vi "PWM Input Post Step.vi"(8 "error in (no error)":errorcluster, 9 "PWM Input In":T1, 10 "Socket No":u16=1, 11 "NI PWM Input in":refnum<class "NI PWM Input.lvclass">) -> (0 "error out":errorcluster, 1 "Frequency":dbl[](array[numeric]), 2 "Report Text":string, 3 "NI PWM Input out":refnum<class "NI PWM Input.lvclass">, 4 "Duty Cycle":dbl[](array[numeric]), 5 "Physical Channel":string[](array[string]))   [LabVIEW 2023, in "HardwareAbstractionLayer_LVOOP.lvlib" / "NI PWM Input.lvclass"]
uses:
  NI PWM Input.lvclass
  Control/PWMInputEdit.ctl
  NI PWM Input.lvclass/NI PWM Input.ctl
  Database/Database.lvclass
  <resource>/objmgr/daqmx.rc
panel:
  out "PhysicalChans":tag[](array[tag])
  out "CounterName":tag[](array[tag])
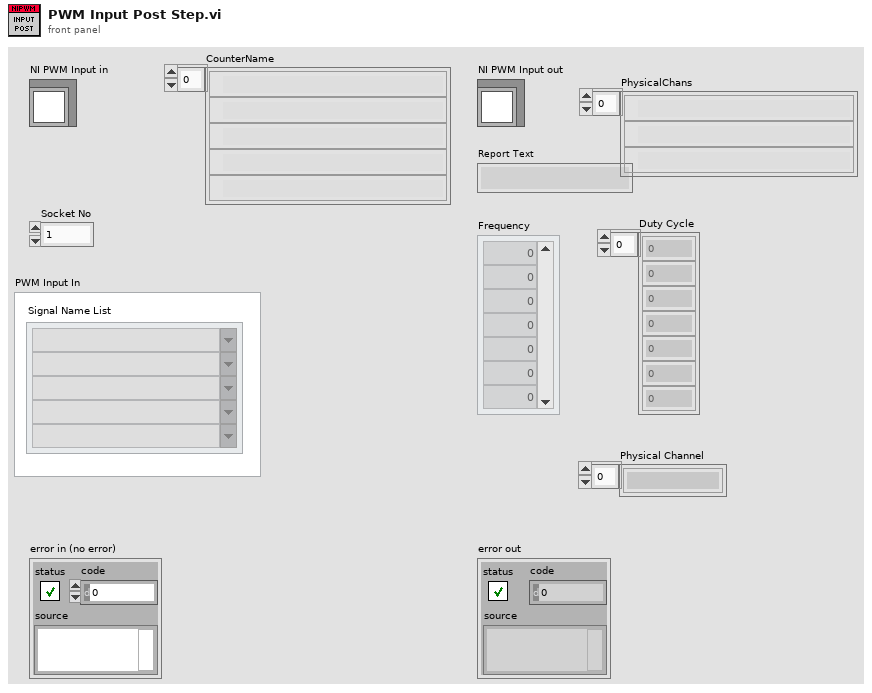
[diagram p1: front panel]
types:
  T1 = typedef "HardwareAbstractionLayer_LVOOP.lvlib/NI PWM Input.lvclass/PWMInputEdit.ctl" = cluster{"Signal Name List":string[]}
  T2 = cluster{"table":string, "condition":string, "columns":string[]}
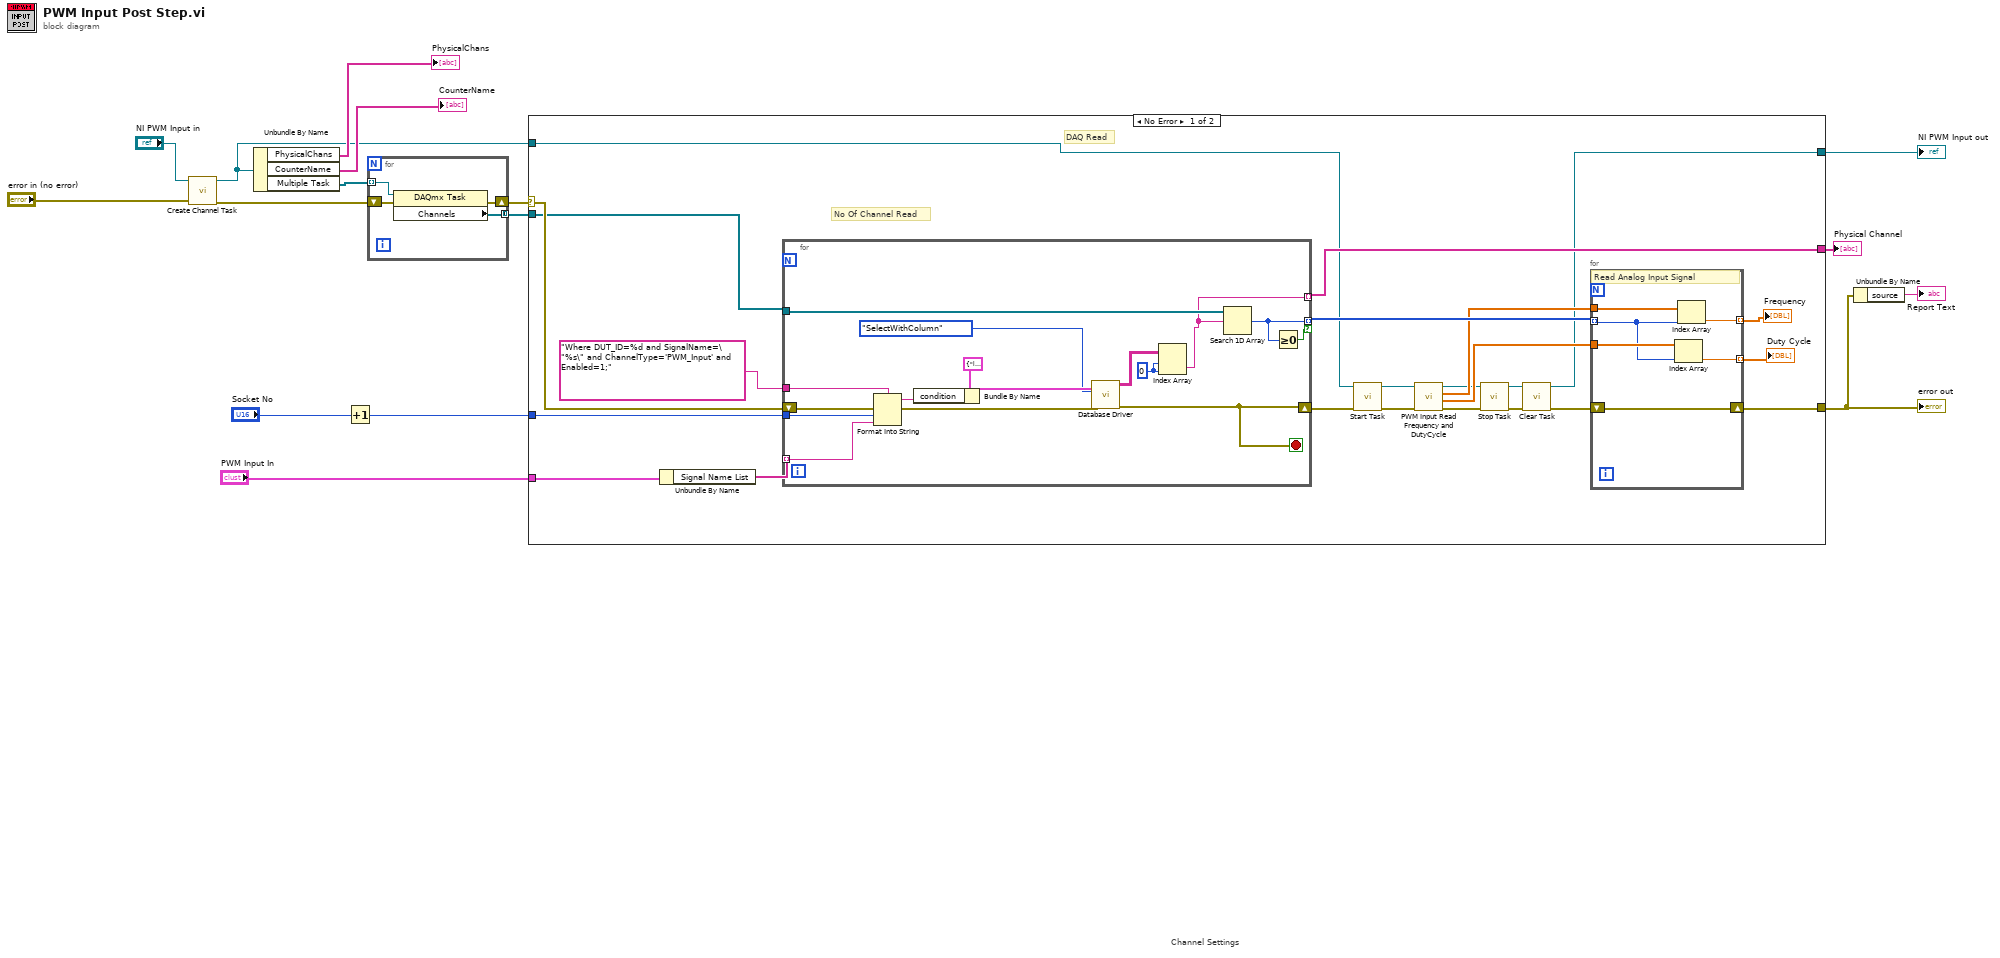
[diagram p0: block diagram]
diagram:
  # "Channel Settings"
  n1 = call-dynamic "Create Channel Task.vi"("error in"="error in (no error)", "NI PWM Input in"="NI PWM Input in") -> ("error out"=w1:errorcluster, "NI PWM Input out"=w3:refnum<class "NI PWM Input.lvclass">)  [unwired: 8 in]
  n2 = Unbundle By Name(w3) -> ("PhysicalChans"=→"PhysicalChans":tag[], "CounterName"=→"CounterName":tag[], "Multiple Task"=w8:refnum<k21>[])
  n3 = Increment(x="Socket No") -> (x+1=w11:u16)
  n4 = for {
    tunnel: [w19] -> w16 mode=concatenating
    shift-right: [w18] -> w10
    shift-left: w1 -> [w20]
    tunnel: w8 -> [w17] mode=indexing
    n5 = property class="DAQmx Task"(reference=w17, error in=w20) -> (error out=w18:errorcluster, "Channels"=w19:refnum<k21>[])  [unwired: 1 out]
  }
  n6 = case shown="No Error" w10 {
    selector: w10 -> [w37 w66]
    tunnel: [w43 w66] -> w13
    tunnel: "PWM Input In" -> [w42 _]
    tunnel: w11 -> [w38 _]
    tunnel: w16 -> [w36 _]
    tunnel: w3 -> [w26 w67]
    tunnel: [w23 w67] -> w14
    tunnel: [w35 _] -> w5
    frame No Error {
      # "No Of Channel Read"
      # "DAQ Read"
      n7 = Unbundle By Name(w42) -> ("Signal Name List"=w41:string[])
      n8 = for {
        tunnel: w41 -> [w57] mode=indexing
        tunnel: "Where DUT_ID=%d and SignalName=\"%s\" and ChannelType='PWM_Input' and Enabled=1;" -> [w59]
        tunnel: w38 -> [w58]
        shift-right: [w47] -> w25
        shift-left: w37 -> [w53]
        tunnel: [w49] -> w39 mode=indexing if=w48
        tunnel: w36 -> [w45]
        tunnel: [w44] -> w35 mode=indexing
        stop <- w47 stop-if-true
        w50 = 0 ("disabled index (col)")
        n9 = Format Into String(format string=w59, error in=w53, w58, w57) -> (resulting string=w55:string, error out=w52:errorcluster)  [unwired: 1 in]
        n10 = Bundle By Name(cluster=T2 {"table"="ltt.daq_configuration", "condition"="Where ChannelType='Analog_Input' and Enabled=1", "columns"=["CounterName"]} ("SQLTableData"), "condition"=w55) -> (w54:T2)
        n11 = call "Database Driver.vi"("SQLTableData"=w54, "error in"=w52, "Select"=enum16{"SelectWithQuery", "SelectWithColumn"}."SelectWithColumn") -> ("error out"=w47:errorcluster, "data"=w51:string[][])  [unwired: 5 in, 2 out]
        n12 = Index Array(array=w51, index (row)=w50, index (col)=w50) -> (element=w44:string)
        n13 = Search 1D Array(1D array=w45, element=w44) -> (index of element=w49:i32)  [unwired: 1 in]
        n14 = Greater Or Equal To 0?(x=w49) -> (x >= 0?=w48:bool)
      }
      n15 = call-dynamic "Start Task.vi"("error in"=w25, "NI PWM Input in"=w26) -> ("error out"=w31:errorcluster, "NI PWM Input out"=w32:refnum<class "NI PWM Input.lvclass">)  [unwired: 8 in]
      n16 = call-dynamic "PWM Input Read Frequency and DutyCycle.vi"("error in (no error)"=w31, "NI PWM Input in"=w32) -> ("error out"=w30:errorcluster, "Duty Cycle"=w33:dbl[], "Frequency"=w34:dbl[], "NI PWM Input out"=w29:refnum<class "NI PWM Input.lvclass">)  [unwired: 6 in]
      n17 = call-dynamic "Stop Task.vi"("error in"=w30, "NI PWM Input in"=w29) -> ("error out"=w22:errorcluster, "NI PWM Input out"=w24:refnum<class "NI PWM Input.lvclass">)  [unwired: 8 in]
      n18 = call-dynamic "Clear Task.vi"("error in"=w22, "NI PWM Input in"=w24) -> ("error out"=w21:errorcluster, "NI PWM Input out"=w23:refnum<class "NI PWM Input.lvclass">)  [unwired: 8 in]
      n19 = for {
        shift-right: [w65] -> w43
        shift-left: w21 -> [w65]
        tunnel: w34 -> [w64]
        tunnel: w39 -> [w61] mode=indexing
        tunnel: [w63] -> w27 mode=indexing
        tunnel: w33 -> [w62]
        tunnel: [w60] -> w28 mode=indexing
        # "Read Analog Input Signal"
        n20 = Index Array(array=w62, index=w61) -> (element=w60:dbl)
        n21 = Index Array(array=w64, index=w61) -> (element=w63:dbl)
      }
      "Frequency" <- w27
      "Duty Cycle" <- w28
    }
    frame Error {
    }
  }
  "error out" <- w13
  "NI PWM Input out" <- w14
  "Physical Channel" <- w5
  n22 = Unbundle By Name(w13) -> ("source"=→"Report Text":string)
